vi "ReadSizeMat_Anything.vi"(8 "error in":errorcluster, 11 "Datatype":refnum<class "Anything.lvclass">) -> (0 "error out":errorcluster, 1 "Height":i32, 2 "Width":i32, 3 "Datatype":refnum<class "Anything.lvclass">, 4 "Channel":i32)   [LabVIEW 2020, in "OpenLvVision_OpenCv.lvlib"]
doc: "Read size of the datatype\nNo malleable to breake vi inlining!"
uses:
  OpenLvVision_OpenCv.lvlib
  Anything.lvclass
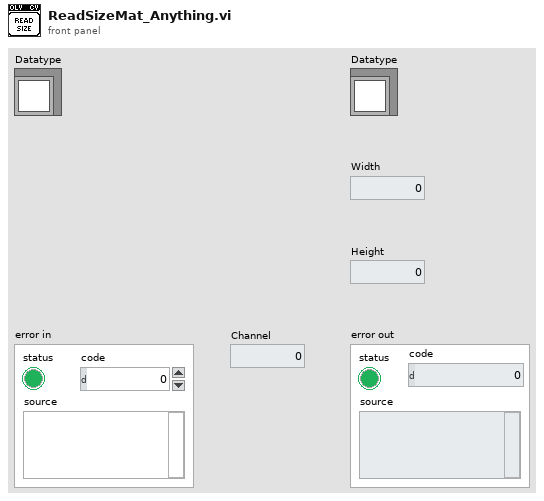
[diagram p1: front panel]
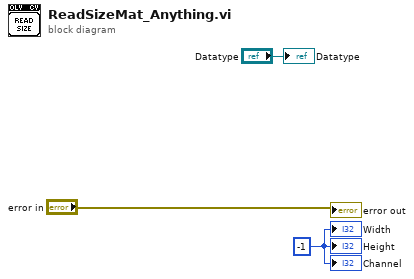
[diagram p0: block diagram]
diagram:
  w1 = -1
  "error out" <- "error in"
  "Width" <- w1
  "Height" <- w1
  "Channel" <- w1
  "Datatype" <- "Datatype"
